vi "Get Setting Folder Path.vi"(8 "error in (no error)":errorcluster, 11 "LabVIEW Object in":refnum<class>) -> (0 "error out":errorcluster, 2 "appended path":path, 3 "LabVIEW Object out":refnum<class>)   [LabVIEW 2023, in "Label-Driven UI.lvlib"]
uses:
  Label-Driven UI.lvlib
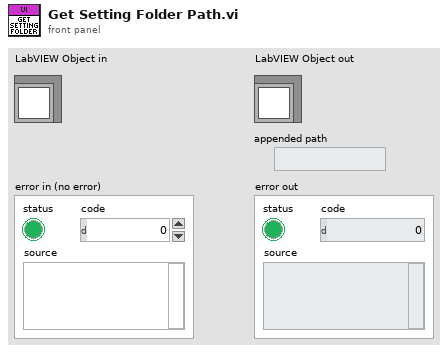
[diagram p1: front panel]
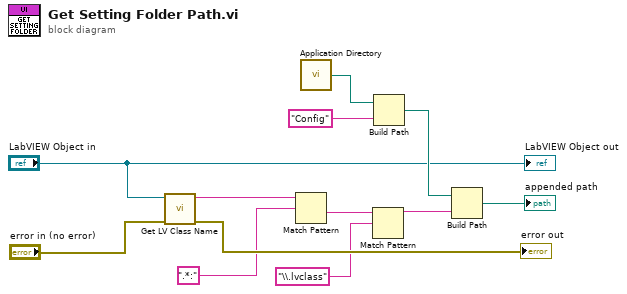
[diagram p0: block diagram]
diagram:
  n1 = call <vilib>:"Get LV Class Name.vi"("error in (no error)"="error in (no error)", "object"="LabVIEW Object in") -> ("error out"=→"error out":errorcluster, "class name"=w2:string)  [unwired: 8 in]
  n2 = Match Pattern(string=w2, regular expression=".*:") -> (after substring=w4:string)  [unwired: 1 in, 3 out]
  n3 = call <vilib>:"Application Directory.vi"() -> ("Application Directory"=w7:path)
  n4 = Match Pattern(string=w4, regular expression="\\.lvclass") -> (before substring=w10:string)  [unwired: 1 in, 3 out]
  n5 = Build Path(base path=w7, name or relative path="Config") -> (appended path=w9:path)
  n6 = Build Path(base path=w9, name or relative path=w10) -> (appended path=→"appended path":path)
  "LabVIEW Object out" <- "LabVIEW Object in"
